vi "PM5000_VI_Polar.vi"(8 "error in":errorcluster, 11 "Network Path":string="172.22.26.202") -> (0 "error out":errorcluster, 1 "VI_Polar_array":sgl[](array[numeric]), 2 "VI_polar out":T1, 3 "Network Path out":string="192.168.169.1")   [LabVIEW 2018]
doc: "Lee la tabla de memoria RealTime_VIF_Power del equipo PowerMonitor 5000, ademas filtra y ordena las variables de interez de la tabla de memoria.\n\nLee las siguientes variables de la tabla RealTime_VIF_Power:\n\n*V1_V2_Volts\n*V2_V3_Volts\n*V3_V1_Volts\n*I1_Amps\n*I2_Amps\n*I3_Amps\n*Frequency_Hz\n*Total_kW\n*Total_kVAR\n*Total_kVA\n*Total_True_PF\n*Total_Disp_PF"
uses:
  <vilib>/ethernetip/ethernetip.llb/EthernetIP SLC500 Read Float.vi
  <vilib>/ethernetip/ethernetip.lvlib
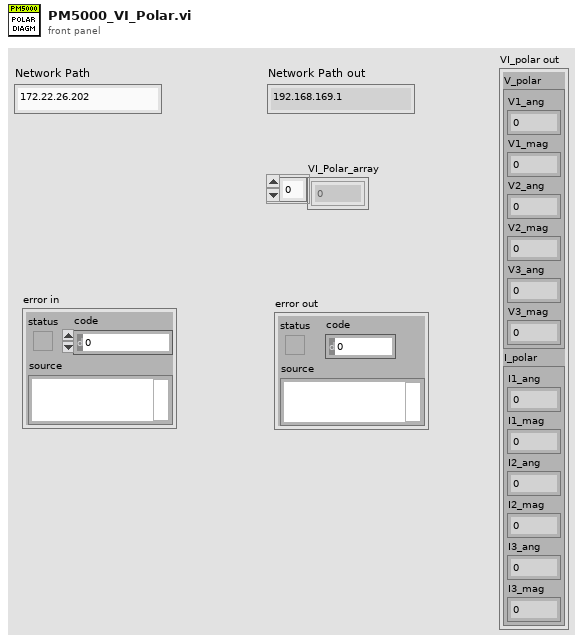
[diagram p1: front panel]
types:
  T1 = cluster{"V_polar":cluster{"V1_ang":sgl, "V1_mag":sgl, "V2_ang":sgl, "V2_mag":sgl, "V3_ang":sgl, "V3_mag":sgl}, "I_polar":cluster{"I1_ang":sgl, "I1_mag":sgl, "I2_ang":sgl, "I2_mag":sgl, "I3_ang":sgl, "I3_mag":sgl}}
  T2 = cluster{"I1_ang":sgl, "I1_mag":sgl, "I2_ang":sgl, "I2_mag":sgl, "I3_ang":sgl, "I3_mag":sgl}
  T3 = cluster{"V1_ang":sgl, "V1_mag":sgl, "V2_ang":sgl, "V2_mag":sgl, "V3_ang":sgl, "V3_mag":sgl}
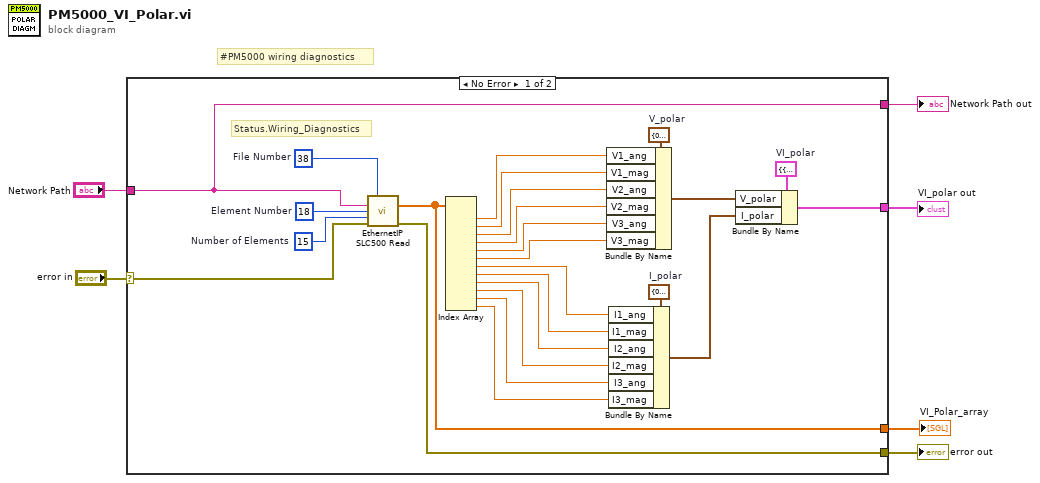
[diagram p0: block diagram]
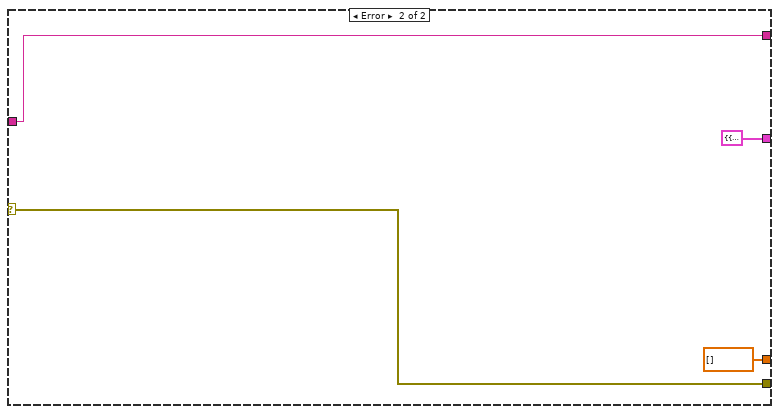
[diagram p2: hidden frame]
diagram:
  # "#PM5000 wiring diagnostics"
  n1 = case shown="No Error" "error in" {
    selector: "error in" -> [w28 w34]
    tunnel: [w10 T1 {"V_polar"={"V1_ang"=0.0, "V1_mag"=0.0, "V2_ang"=0.0, "V2_mag"=0.0, "V3_ang"=0.0, "V3_mag"=0.0}, "I_polar"={"I1_ang"=0.0, "I1_mag"=0.0, "I2_ang"=0.0, "I2_mag"=0.0, "I3_ang"=0.0, "I3_mag"=0.0}} ("VI_polar")] -> w5
    tunnel: [w7 w32] -> w4
    tunnel: [w9 w34] -> w3
    tunnel: [w8 sgl[] [] ("Data")] -> w2
    tunnel: "Network Path" -> [w7 w32]
    frame No Error {
      w25 = T2 {"I1_ang"=0.0, "I1_mag"=0.0, "I2_ang"=0.0, "I2_mag"=0.0, "I3_ang"=0.0, "I3_mag"=0.0}  # I_polar
      w24 = T3 {"V1_ang"=0.0, "V1_mag"=0.0, "V2_ang"=0.0, "V2_mag"=0.0, "V3_ang"=0.0, "V3_mag"=0.0}  # V_polar
      w23 = T1 {"V_polar"={"V1_ang"=0.0, "V1_mag"=0.0, "V2_ang"=0.0, "V2_mag"=0.0, "V3_ang"=0.0, "V3_mag"=0.0}, "I_polar"={"I1_ang"=0.0, "I1_mag"=0.0, "I2_ang"=0.0, "I2_mag"=0.0, "I3_ang"=0.0, "I3_mag"=0.0}}  # VI_polar
      w29 = u32 15  # Number of Elements
      w31 = u16 38  # File Number
      w30 = u16 18  # Element Number
      # "Status.Wiring_Diagnostics"
      n2 = call-poly <vilib>:"EthernetIP SLC500 Read.vi"("File Number"=w31, "Network Path"=w7, "Element Number"=w30, "Number of Elements"=w29, "error in"=w28) -> ("Data"=w8:sgl[], "error out"=w9:errorcluster)  [unwired: 8 in, 1 out]
      n3 = Index Array(array=w8) -> (element #1=w22:sgl, element #2=w21:sgl, element #3=w20:sgl, element #4=w19:sgl, element #5=w18:sgl, element #6=w17:sgl, element #7=w16:sgl, element #8=w15:sgl, element #9=w14:sgl, element #10=w13:sgl, element #11=w12:sgl, element #12=w11:sgl)  [unwired: 12 in]
      n4 = Bundle By Name(cluster=w24, "V1_ang"=w22, "V1_mag"=w21, "V2_ang"=w20, "V2_mag"=w19, "V3_ang"=w18, "V3_mag"=w17) -> (w26:T3)
      n5 = Bundle By Name(cluster=w25, "I1_ang"=w16, "I1_mag"=w15, "I2_ang"=w14, "I2_mag"=w13, "I3_ang"=w12, "I3_mag"=w11) -> (w27:T2)
      n6 = Bundle By Name(cluster=w23, "V_polar"=w26, "I_polar"=w27) -> (w10:T1)
    }
    frame Error {
    }
  }
  "error out" <- w3
  "Network Path out" <- w4
  "VI_polar out" <- w5
  "VI_Polar_array" <- w2
